vi "OutputChannelSignalSet.vi"(0 "SR865 in":T3, 2 "OutputChannel":T2 caption="Output channel" items=["Channel 1", "Channel 2"], 3 "OutputChannelSignal":T1 caption="Output channel signal" items=["X (ch1) / Y (ch2)", "R (ch1) / Q (ch2)"], 5 "error in":errorcluster) -> (14 "SR865 out":T3, 19 "error out":errorcluster)   [LabVIEW 2017]
uses:
  SR865.ctl
  OutputChannel.ctl
  OutputChannelSignal.ctl
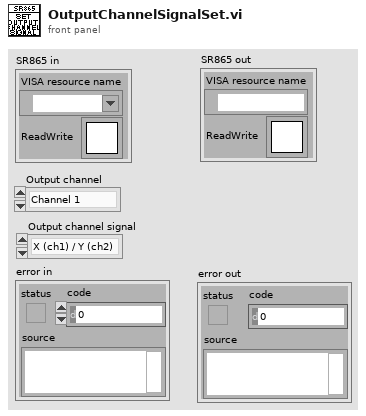
[diagram p1: front panel]
types:
  T1 = typedef "OutputChannelSignal.ctl" = u16
  T2 = typedef "OutputChannel.ctl" = u16
  T3 = typedef "SR865.ctl" = cluster{"VISA resource name":refnum<visa-resource-name>, "ReadWrite":T4}
  T4 = typedef "Semaphore RefNum" = refnum<k1>
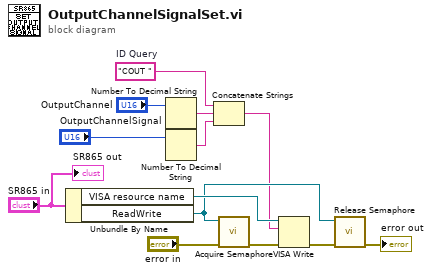
[diagram p0: block diagram]
diagram:
  w7 = "COUT "  # ID Query
  n1 = Unbundle By Name("SR865 in") -> ("VISA resource name"=w12:refnum<visa-resource-name>, "ReadWrite"=w8:T4)
  n2 = Number To Decimal String(number="OutputChannel") -> (decimal integer string=w5:string)  [unwired: 1 in]
  n3 = Number To Decimal String(number="OutputChannelSignal") -> (decimal integer string=w2:string)  [unwired: 1 in]
  n4 = Concatenate Strings(w7, w5, w2) -> (w4:string)
  n5 = call <vilib>:"Acquire Semaphore.vi"("error in (no error)"="error in", "semaphore"=w8) -> ("error out"=w11:errorcluster)  [unwired: 3 in, 2 out]
  n6 = VISA Write(VISA resource name=w12, write buffer=w4, error in (no error)=w11) -> (error out=w3:errorcluster)  [unwired: 2 out]
  n7 = call <vilib>:"Release Semaphore.vi"("error in (no error)"=w3, "semaphore"=w8) -> ("error out"=→"error out":errorcluster)  [unwired: 4 in, 1 out]
  "SR865 out" <- "SR865 in"
